vi "PCO_AllocateBuffer.vi"(8 "error in (no error)":errorcluster, 9 "dwSize (words)":u32=1447680, 10 "sBufNr":i16=-1, 11 "Handle":u32=136659496) -> (0 "error out":errorcluster, 1 "words allocated":u32, 2 "sBufNr out":i16, 3 "Handle Out":u32=136659496, 4 "wBuf":u16[](array[numeric]), 5 "return type":u32 format="%x")   [LabVIEW 2011]
panel:
  # "This does not work!!!!\narray handle crashes\narray handle pointer also crashes"
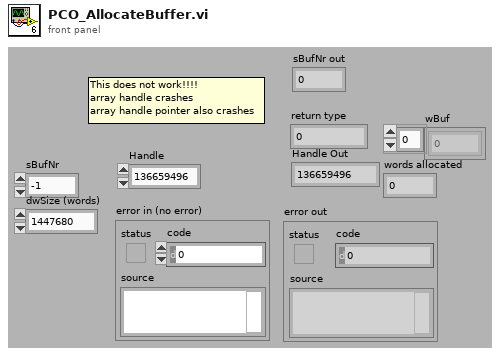
[diagram p1: front panel]
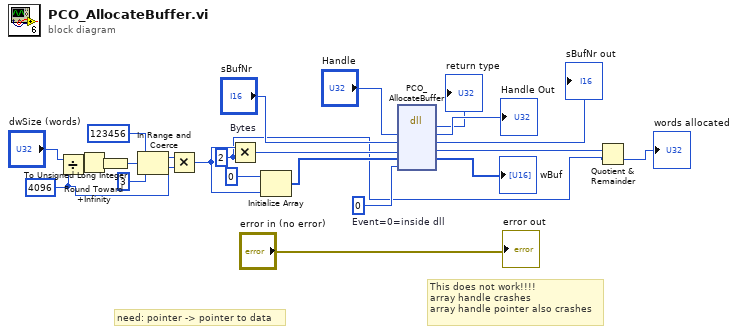
[diagram p0: block diagram]
diagram:
  w1 = u32 2 ("y")
  w5 = u32 4096 ("y")
  w19 = 0  # Event=0=inside dll
  # "need: pointer -> pointer to data"
  # "This does not work!!!!\narray handle crashes\narray handle pointer also crashes"
  n1 = Divide(x="dwSize (words)", y=w5) -> (x/y=w13:dbl)
  n2 = Round Toward +Infinity(x=w13) -> (ceil(x): smallest int >= x=w12:dbl)
  n3 = To Unsigned Long Integer(number=w12) -> (unsigned 32bit integer=w11:u32)
  n4 = In Range and Coerce(upper limit=u32 123456, x=w11, lower limit=u32 3) -> (coerced(x)=w8:u32)  [unwired: 1 out]
  n5 = Multiply(x=w8, y=w5) -> (x*y=w6:u32)
  n6 = Multiply "Bytes"(x=w6, y=w1) -> (x*y=w4:u32)
  n7 = Initialize Array(u16 0, w6) -> (w16:u16[])
  n8 = dll-call lib="?" fn="PCO_AllocateBuffer"("Handle"="Handle", "sBufNr"="sBufNr", "dwSize"=w4, "wBuf"=w16, "hEvent"=w19) -> ("return type"=→"return type":u32, "Handle"=→"Handle Out":u32, "sBufNr"=→"sBufNr out":i16, "dwSize"=w2:u32, "wBuf"=→"wBuf":u16[])  [unwired: 3 in, 3 out]
  n9 = Quotient & Remainder(x=w2, y=w1) -> (floor(x/y)=→"words allocated":u32)  [unwired: 1 out]
  "error out" <- "error in (no error)"
